vi "compare versions.vi"(9 "VersionNumber 2":T1, 10 "VersionNumber 1":T1) -> (1 "2>1":bool, 2 "1>2":bool, 3 "1=2":bool)   [LabVIEW 2018, in "LV2Julia_core.lvlib"]
uses:
  LV2Julia_core.lvlib
  VersionNumber.ctl
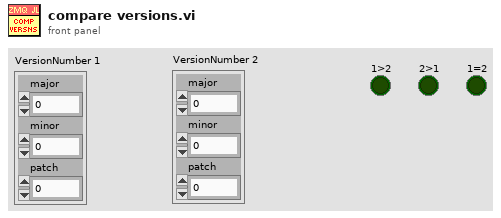
[diagram p1: front panel]
types:
  T1 = typedef "LV2Julia_core.lvlib/VersionNumber.ctl" = cluster{"major":u16, "minor":u16, "patch":u16}
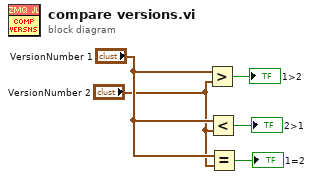
[diagram p0: block diagram]
diagram:
  n1 = Greater?(x="VersionNumber 1", y="VersionNumber 2") -> (0:→"1>2":bool)
  n2 = Less?(x="VersionNumber 1", y="VersionNumber 2") -> (x < y?=→"2>1":bool)
  n3 = Equal?(x="VersionNumber 1", y="VersionNumber 2") -> (x = y?=→"1=2":bool)
